vi "Read Control Experiment.json.vi"(8 "error in (no error)":errorcluster, 10 "file (use dialog)":path, 11 "Control Experiment in":refnum<class "Control Experiment.lvclass">) -> (0 "error out":errorcluster, 2 "output cluster":T1, 3 "Control Experiment out":refnum<class "Control Experiment.lvclass">)   [LabVIEW 2019, in "Control Experiment.lvclass"]
uses:
  Control Experiment.lvclass
  Typedefs/Control Experiment JSON--cluster.ctl
  6bb5f8be-f1e2-427f-a6d8-5173d26fd901.vi
  <vilib>/JDP Science/JSONtext/JSON text to Variant.vi
  <vilib>/JDP Science/JSONtext/LVClass Serializer/JSONtext LVClass Serializer.lvclass
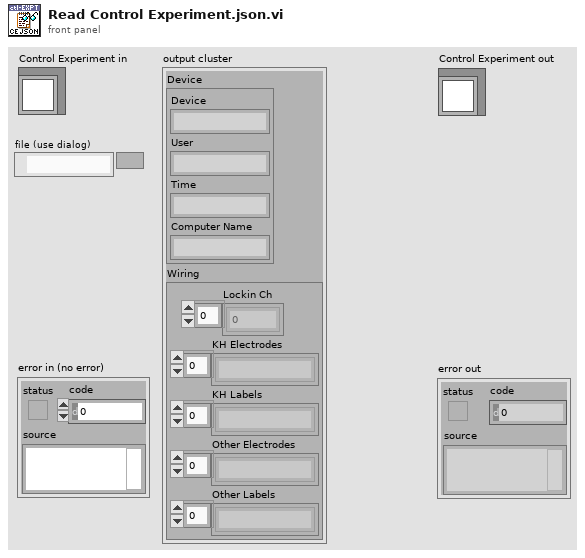
[diagram p1: front panel]
types:
  T1 = typedef "Control Experiment.lvclass/Control Experiment JSON--cluster.ctl" = cluster{"Device":cluster{"Device":string, "User":string, "Time":string, "Computer Name":string}, "Wiring":cluster{"Lockin Ch":u32[], "KH Electrodes":string[], "KH Labels":string[], "Other Electrodes":string[], "Other Labels":string[]}}
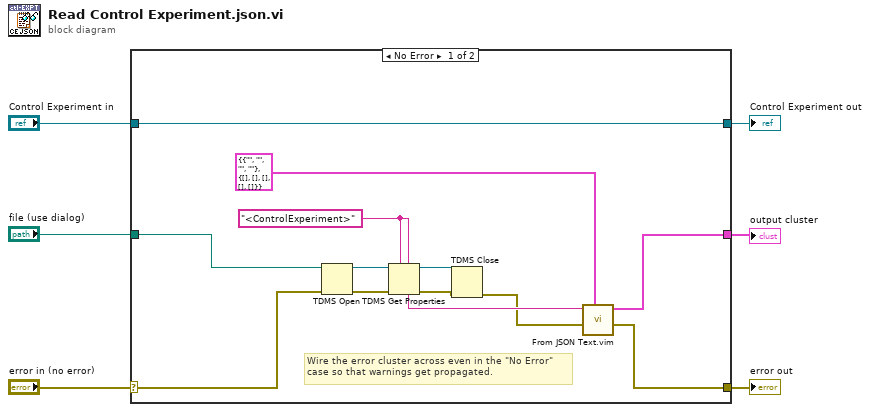
[diagram p0: block diagram]
diagram:
  n1 = case shown="No Error" "error in (no error)" {
    selector: "error in (no error)" -> [w14 w21]
    tunnel: [w9 w21] -> w5
    tunnel: [w19 w20] -> w3
    tunnel: "Control Experiment in" -> [w19 w20]
    tunnel: "file (use dialog)" -> [w13 _]
    tunnel: [w10 _] -> w1
    frame No Error {
      w18 = "<ControlExperiment>" ("group name")
      # "Wire the error cluster across even in the \"No Error\"\ncase so that warnings get propagated."
      n2 = TDMS Open(8:w14, 11:w13) -> (0:w12:errorcluster, 3:w17:refnum<k34>)  [unwired: 5 in]
      n3 = TDMS Get Properties(5:w18, 7:w18, 8:w12, 11:w17) -> (0:w11:errorcluster, 3:w16:refnum<k34>, 4:w15:string)  [unwired: 2 in, 3 out]
      n4 = TDMS Close(8:w11, 11:w16) -> (0:w8:errorcluster)  [unwired: 1 out]
      n5 = call "From JSON Text.vim"("Data Type and Default Value"=T1 {"Device"={"Device"="", "User"="", "Time"="", "Computer Name"=""}, "Wiring"={"Lockin Ch"=[], "KH Electrodes"=[], "KH Labels"=[], "Other Electrodes"=[], "Other Labels"=[]}} ("output cluster"), "error in (no error)"=w8, "JSON"=w15) -> ("error out"=w9:errorcluster, "Data out"=w10:T1)  [unwired: 7 in]
    }
    frame Error {
    }
  }
  "error out" <- w5
  "Control Experiment out" <- w3
  "output cluster" <- w1
